vi "XLP80_CAN_GetReadIndex.vi"(6 "Init":bool, 10 "CAN Read Items":T1=enum."C_07_BAT_s_SoC") -> (2 "Index":i32)   [LabVIEW 2021]
uses:
  XLP80_FGlob/1886_FGlob_TDefEnumCANReadItems.ctl
  XLP80_Globals/XLP80_Globals_Status.vi
  XLP80_Globals/Globals_Settings_XLP80.vi
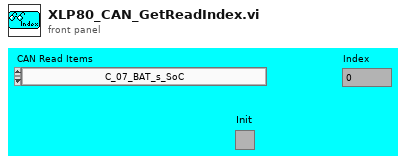
[diagram p1: front panel]
types:
  T1 = typedef "1886_FGlob_TDefEnumCANReadItems.ctl" = enum16{"A03_ETC_a_opCmd1_Start_Stop", "A03_ETC_s_Speed_Actual", "A11_HBV_s_Valve_Act", "A12_SIV_s_Valve_Act", "A13_SOV_s_Valve_Act", "A14_HFM_s_AirMassFlow", "A14_HFM_s_Humidity", "A14_HFM_s_Pressure", "A14_HFM_s_Temperature", "A15_SI_s_Inlet_Pressure", "A15_SI_s_Inlet_Pressure_FM12", "A15_SI_s_Inlet_Temperature", "A16_SI_s_Inlet_Temperature", "A17_SO_s_Outlet_Pressure", "A17_SO_s_Outlet_Pressure_FM12", "A17_SO_s_Outlet_Temperature", "A22_HSI_s_Humidity", "A22_HSI_s_Humidity_FM12", "A23_HSO_s_Humidity", "A56_SO_s_Temperature", "C01_RF_a_FanSpeed", "C02_CP_s_ACTUAL_SPEED_FM2", "C02_CP_a_ENABLE_FM2", "C02_CP_a_RPM", "C04_DI_s_Temperature", "C06_ET_s_CoolLevelStatus", "C07_BAT_s_Board_Temperature", "C07_BAT_s_External_Load_Voltage", "C_07_BAT_s_SoC", "C07_BAT_s_System_Current", "C08_AMB_s_Humidity_Rel", "C08_AMB_s_Pressure", "C08_AMB_s_Temperature", "C24_TRO_s_Temperature_FM23", "C27_RIV_a_Valve_Set_FM2", "C28_RBV_a_Valve_Set_FM2", "C29_TSO_s_Temperature_FM3", "C54_SI_s_Temperature", "C61_SV_a_FanEnable_FM2", "E71_DC4880_s_Current_In_Actual", "E71_DC4880_s_Current_Out_Actual", "E71_DC4880_s_Temperature_1_Act", "E71_DC4880_s_Voltage_Out_Actual", "E71_DC4880_s_Voltage_In_Actual", "E76_HVM_a_Relais_Set", "E75_HVP_a_Relais_Set", "H31_OTV_a_Valve_Set", "H_31_OTV_s_Pressure", "H31_OTV_s_Pressure_FM12", "H_31_OTV_s_Temperature", "H36_GHU_s_Pressure_1", "H36_GHU_s_Pressure_1_FM12", "H37_GHU_s_Temperature_1", "H36_GHU_s_Temperature_FM2", "H38_HSV_a_Valve_Set", "H40_GHU_s_Pressure_2", "H40_GHU_s_Pressure_2_FM12", "H41_GHU_s_Temperature_2", "H42_HRB_s_ARB_Spd", "H43_HDV_a_Dosing_Valve_Set", "H45_WT_s_WaterLevelStatus", "H51_STK_s_CellVolt_highest_2003", "H51_STK_s_CellVolt_lowest_2003", "H51_STK_s_TotalVoltage_2003", "H52_DV_a_Drain_Valve_Stack_Set", "H53_PV_a_Purge_Valve_Stack_Set", "H55_SI_s_Stack_Inlet_Pressure", "H62_HLD_s_H2_Concentration", "H63_HLD_s_H2_Concentration", "H63_HLD_s_concH2_FM2", "S91_SYS_MasterCtrl_State", "S91_SYS_PowerCtrl_State", "S91_SYS_Error_Code", "S91_SYS_Error_Level"}
  T2 = typedef "XLP80_Action_TDefEnumControl.ctl" = enum16{"Testmode_A", "Testmode_B"}
  T3 = cluster{"Signal Name":string[], "Description":string[], "Unit":string[], "Min":dbl[], "Max":dbl[], "TestmodeA":bool[], "LogEnable":bool[]}
  T4 = cluster{"Signal Name":string[], "Description":string[], "Unit":string[], "Min":dbl[], "Max":dbl[], "HV & Software":bool[], "Basis Funktion":bool[], "Power Management":bool[], "OperationMode":bool[], "Shutdown":bool[], "Alarm":bool[], "LogEnable":bool[]}
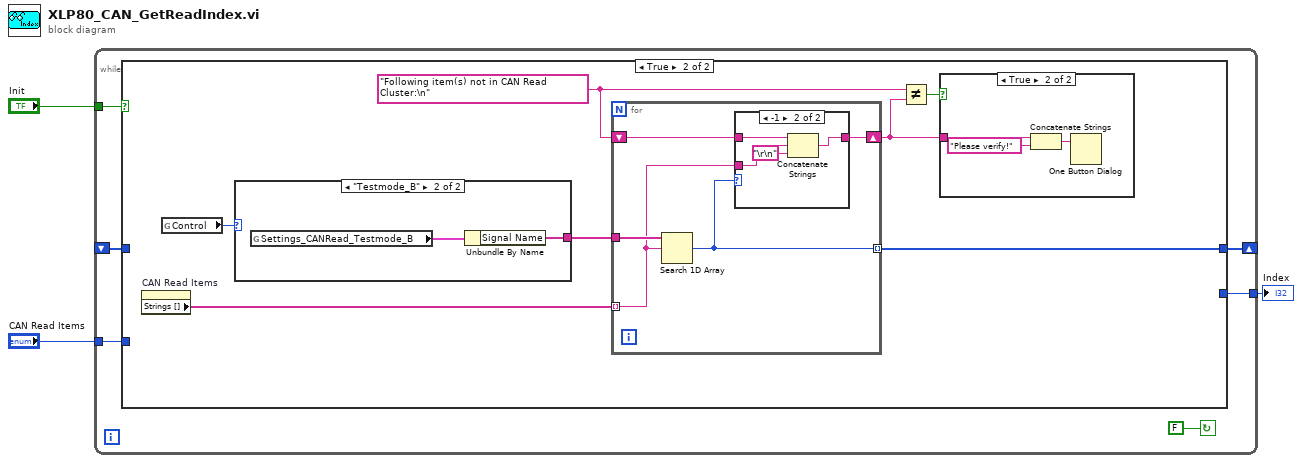
[diagram p0: block diagram]
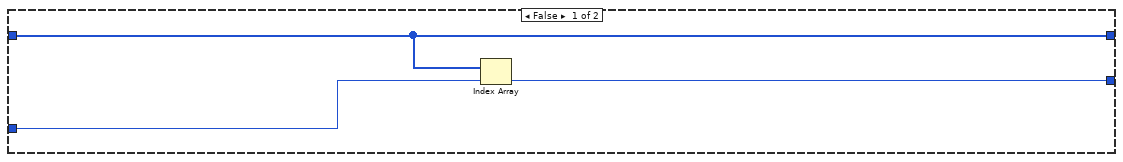
[diagram p2: hidden frame]
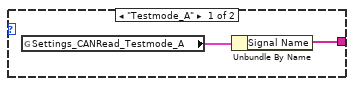
[diagram p5: hidden frame]
diagram:
  n1 = while {
    tunnel: "Init" -> [w8]
    tunnel: "CAN Read Items" -> [w7]
    shift-right: [w6] -> _
    shift-left: _ -> [w5]
    tunnel: [w4] -> w1
    stop <- FALSE continue-if-true
    n2 = case shown="True" w8 {
      tunnel: w7 -> [w11 _]
      tunnel: [w12 w17] -> w6
      tunnel: w5 -> [w12 _]
      tunnel: [w10 _] -> w4
      frame False {
        n3 = Index Array(array=w12, index=w11) -> (element=w10:i32)
      }
      frame True {
        w15 = "Following item(s) not in CAN Read Cluster:\n"
        n4 = property on="CAN Read Items" class="Enum (strict)"() -> ("Strings []"=w16:string[])  [unwired: 2 in, 2 out]
        n5 = global read "XLP80_Globals_Status.vi" "Control"() -> (w19:T2)
        n6 = case shown="\"Testmode_B\"" w19 {
          tunnel: [w33 w35] -> w18
          frame "Testmode_A" {
            n7 = global read "Globals_Settings_XLP80.vi" "Settings_CANRead_Testmode_A"() -> (w34:T3)
            n8 = Unbundle By Name(w34) -> ("Signal Name"=w33:string[])
          }
          frame "Testmode_B" {
            n9 = global read "Globals_Settings_XLP80.vi" "Settings_CANRead_Testmode_B"() -> (w36:T4)
            n10 = Unbundle By Name(w36) -> ("Signal Name"=w35:string[])
          }
        }
        n11 = for {
          tunnel: w18 -> [w27]
          tunnel: [w26] -> w17 mode=indexing
          tunnel: w16 -> [w25] mode=indexing
          shift-right: [w23] -> w13
          shift-left: w15 -> [w24]
          n12 = Search 1D Array(1D array=w27, element=w25) -> (index of element=w26:i32)  [unwired: 1 in]
          n13 = case shown="-1" w26 {
            tunnel: w25 -> [_ w30]
            tunnel: w24 -> [w28 w32]
            tunnel: [w28 w31] -> w23
            frame Default {
            }
            frame -1 {
              n14 = Concatenate Strings(w32, w30, "\r\n") -> (w31:string)
            }
          }
        }
        n15 = Not Equal?(x=w15, y=w13) -> (x != y?=w14:bool)
        n16 = case shown="True" w14 {
          tunnel: w13 -> [_ w22]
          frame False {
          }
          frame True {
            n17 = Concatenate Strings(w22, "Please verify!" ("string")) -> (w21:string)
            n18 = One Button Dialog(message=w21) -> ()  [unwired: 1 in, 1 out]
          }
        }
      }
    }
  }
  "Index" <- w1
